vi "Flashing_Config Parse.vi"(0 "Config File Path":path, 11 "Error In":errorcluster) -> (4 "Pass/Fail?":bool, 6 "Report Text":string, 8 "VALEW_config":T1, 15 "Error Out":errorcluster)   [LabVIEW 2014]
uses:
  Washer/Product Testcode/VALEW/Valew Common/Config/type defs/DryerConfig.ctl
  <vilib>/Utility/config.llb/Read Key (String).vi
  <vilib>/Utility/config.llb/Read Key (Boolean).vi
  <vilib>/Utility/config.llb/NI_LVConfig.lvlib
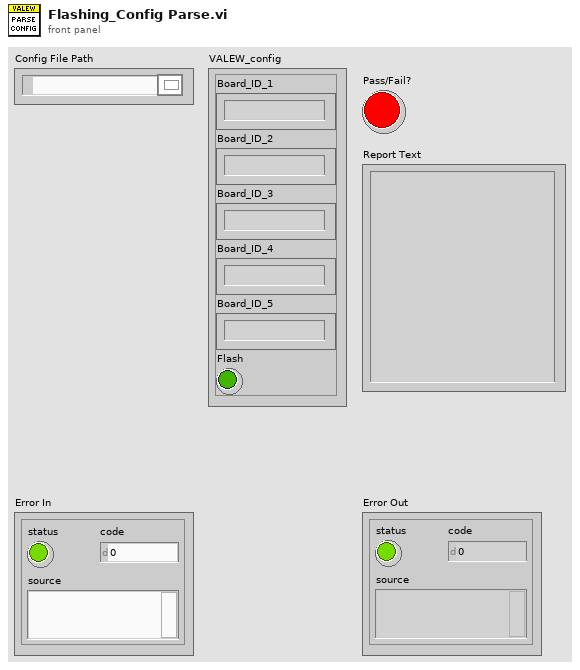
[diagram p1: front panel]
types:
  T1 = typedef "DryerConfig.ctl" = cluster{"Board_ID_1":string, "Board_ID_2":string, "Board_ID_3":string, "Board_ID_4":string, "Board_ID_5":string, "Flash":bool}
  T2 = typedef "NI_LVConfig.lvlib/Config Data RefNum.ctl" = refnum<k1>
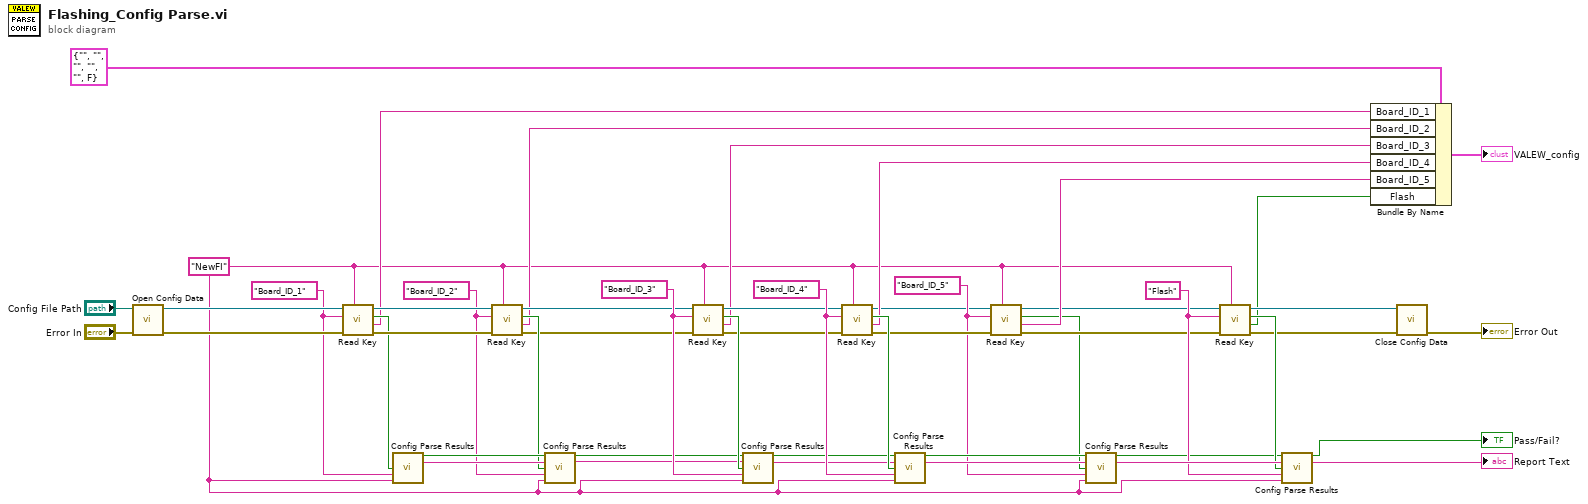
[diagram p0: block diagram]
diagram:
  w9 = "Board_ID_5" ("key")
  w35 = "Board_ID_4" ("key")
  w30 = "Board_ID_3" ("key")
  w36 = "Flash" ("key")
  w39 = "Board_ID_2" ("key")
  w44 = "Board_ID_1" ("key")
  w6 = "NewFI" ("section")
  n1 = call <vilib>:"Open Config Data.vi"("error in (no error)"="Error In", "configuration file path"="Config File Path") -> ("error out"=w47:errorcluster, "refnum"=w48:T2)  [unwired: 7 in, 1 out]
  n2 = call-poly <vilib>:"Read Key.vi"("section"=w6, "error in (no error)"=w47, "key"=w44, "refnum"=w48) -> ("error out"=w49:errorcluster, "value"=w23:string, "found?"=w43:bool, "refnum out"=w50:T2)  [unwired: 4 in]
  n3 = call "Config Parse Results.vi"("found?"=w43, "key"=w44, "section"=w6) -> ("Pass/Fail"=w42:bool, "Report Text"=w41:string)  [unwired: 11 in]
  n4 = call-poly <vilib>:"Read Key.vi"("section"=w6, "error in (no error)"=w49, "key"=w39, "refnum"=w50) -> ("error out"=w27:errorcluster, "value"=w22:string, "found?"=w40:bool, "refnum out"=w28:T2)  [unwired: 4 in]
  n5 = call "Config Parse Results.vi"("Previous Pass/Fail"=w42, "Previous Report Text"=w41, "found?"=w40, "key"=w39, "section"=w6) -> ("Pass/Fail"=w25:bool, "Report Text"=w24:string)  [unwired: 9 in]
  n6 = call-poly <vilib>:"Read Key.vi"("section"=w6, "error in (no error)"=w27, "key"=w30, "refnum"=w28) -> ("error out"=w26:errorcluster, "value"=w21:string, "found?"=w31:bool, "refnum out"=w29:T2)  [unwired: 4 in]
  n7 = call "Config Parse Results.vi"("Previous Pass/Fail"=w25, "Previous Report Text"=w24, "found?"=w31, "key"=w30, "section"=w6) -> ("Pass/Fail"=w32:bool, "Report Text"=w33:string)  [unwired: 9 in]
  n8 = call-poly <vilib>:"Read Key.vi"("section"=w6, "error in (no error)"=w26, "key"=w35, "refnum"=w29) -> ("error out"=w11:errorcluster, "value"=w20:string, "found?"=w34:bool, "refnum out"=w4:T2)  [unwired: 4 in]
  n9 = call "Config Parse Results.vi"("Previous Pass/Fail"=w32, "Previous Report Text"=w33, "found?"=w34, "key"=w35, "section"=w6) -> ("Pass/Fail"=w19:bool, "Report Text"=w18:string)  [unwired: 9 in]
  n10 = call-poly <vilib>:"Read Key.vi"("section"=w6, "error in (no error)"=w11, "key"=w9, "refnum"=w4) -> ("error out"=w10:errorcluster, "value"=w8:string, "found?"=w1:bool, "refnum out"=w3:T2)  [unwired: 4 in]
  n11 = call "Config Parse Results.vi"("Previous Pass/Fail"=w19, "Previous Report Text"=w18, "found?"=w1, "key"=w9, "section"=w6) -> ("Pass/Fail"=w2:bool, "Report Text"=w38:string)  [unwired: 9 in]
  n12 = call-poly <vilib>:"Read Key.vi"("section"=w6, "error in (no error)"=w10, "key"=w36, "refnum"=w3) -> ("error out"=w12:errorcluster, "value"=w7:bool, "found?"=w37:bool, "refnum out"=w13:T2)  [unwired: 4 in]
  n13 = call "Config Parse Results.vi"("Previous Pass/Fail"=w2, "Previous Report Text"=w38, "found?"=w37, "key"=w36, "section"=w6) -> ("Pass/Fail"=→"Pass/Fail?":bool, "Report Text"=→"Report Text":string)  [unwired: 9 in]
  n14 = Bundle By Name(cluster=T1 {"Board_ID_1"="", "Board_ID_2"="", "Board_ID_3"="", "Board_ID_4"="", "Board_ID_5"="", "Flash"=FALSE} ("VALEW_config"), "Board_ID_1"=w23, "Board_ID_2"=w22, "Board_ID_3"=w21, "Board_ID_4"=w20, "Board_ID_5"=w8, "Flash"=w7) -> (→"VALEW_config":T1)
  n15 = call <vilib>:"Close Config Data.vi"("error in (no error)"=w12, "refnum"=w13) -> ("error out"=→"Error Out":errorcluster)  [unwired: 8 in, 1 out]
